vi "Load data into Tree.vi"(8 "error in (no error)":errorcluster, 11 "Execution UI In":refnum<class "Execution UI V2.lvclass">) -> (0 "error out":errorcluster, 3 "Execution UI Out":refnum<class "Execution UI V2.lvclass">)   [LabVIEW 2020]
uses:
  Execution UI V2.lvclass
  Execution UI V2.lvclass/Execution UI V2.ctl
  Framework/Helper Classes/Test Finder/Test Finder.lvclass/Test Finder.ctl
  Framework/Helper Classes/Result Table/Result Table/Result Table.lvclass/Result Table.ctl
  Framework/Helper Classes/Test Result Tree/Test Result Tree.lvclass
  C:/Git/astemes-lunit/source/Framework/Helper Classes/Test Tree/Test Tree.lvclass
  Framework/Helper Classes/Test Finder/Public/Accessors/Read Test Method Names.vi
  Framework/Helper Classes/Test Tree/Test Tree.lvclass
  Framework/Helper Classes/Result Table/Result Table/Result Table.lvclass
  C:/Git/astemes-lunit/source/Framework/Helper Classes/Test Result Tree/Test Result Tree.lvclass
  C:/Git/astemes-lunit/source/Application Framework/Process Classes/Process/Process.lvclass
  C:/Git/astemes-lunit/source/Rewrite Project/Execution UI/Execution UI V2.lvclass
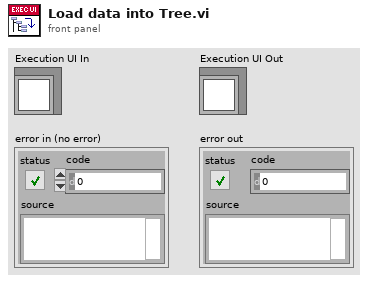
[diagram p1: front panel]
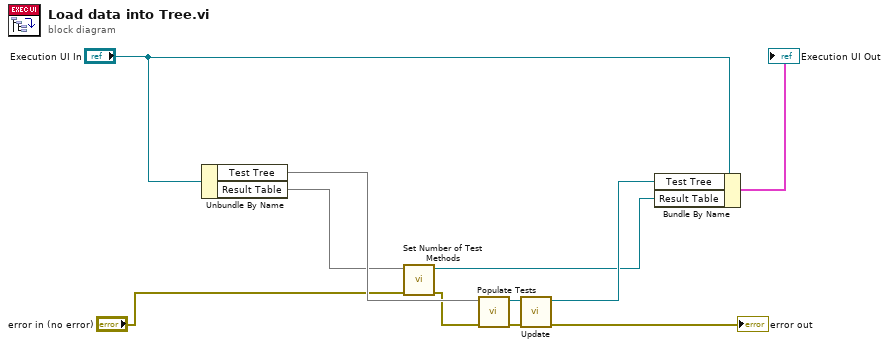
[diagram p0: block diagram]
diagram:
  n1 = Unbundle By Name("Execution UI In") -> ("Test Tree"=w7, "Result Table"=w4)
  n2 = call "Set Number of Test Methods.vi"("error in (no error)"="error in (no error)", "Result Table.lvclass"=w4) -> ("error out"=w2:errorcluster, "Result Table"=w1:refnum<class "Result Table.lvclass">)  [unwired: 8 in]
  n3 = call "Populate Tests.vi"("error in (no error)"=w2, "Test Tree In"=w7) -> ("error out"=w5:errorcluster, "Test Tree Out"=w6:refnum<class "Test Result Tree.lvclass">)  [unwired: 7 in, 1 out]
  n4 = call "Update.vi"("error in (no error)"=w5, "Test Tree In"=w6) -> ("error out"=→"error out":errorcluster, "Test Tree Out"=w8:refnum<class "Test Result Tree.lvclass">)  [unwired: 8 in]
  n5 = Bundle By Name(cluster="Execution UI In", "Test Tree"=w8, "Result Table"=w1) -> (→"Execution UI Out":cluster{})
